vi "test_DL950.vi"() -> ()   [LabVIEW 2019]
uses:
  _ctrl/fgv_DL950.ctl
  _ctrl/rw.ctl
  _ctrl/init-r-stop.ctl
  _ctrl/create-rw-close.ctl
  _ctrl/DL950_config.ctl
panel:
  out "DL950 wfm":waveform(dbl)[](graph)
  out "Waveform":cluster{"l":dbl, "dt":dbl, "Y":dbl[][]}(graph)
  out "n":i32
  out "Read":string
  in  "Qurery":bool
  in  "Write":string
  in  "Disconnection":bool
  in  "Connection":bool
  in  "Get_Items":bool
  in  "Get_Wave":bool
  in  "config":T1={"Timeout"=10000, "Time Div"=12, "Acq Mode"=0, "Record Len"=0, "Record Num"=0, "Start Point"=0, "End Poin"=1000, "Visa"="", "Config Voltage"=[], "Trigger on"=FALSE, "Trigger Level"=0.0, "Reset"=FALSE, "Config Temp"=[], "Trigger Mode"=1, "Trigger Position"=50.0, "Trigger Slope"=0, "Trigger Source "=1, "Start Point (-5.00)"=-5.0, "End Point (5.00)"=5.0} {"End Point (5.00)" format="%.2g"; "Start Point (-5.00)" format="%.2f"; "Trigger Source" items=["", "CH1", "CH2", "CH3", "CH4", "CH5", "CH6", "CH7", "CH8", "CH9", "CH10", "CH11", "CH12", "CH13", "CH14", "CH15", "CH16", "RMATH1", "RMATH2", "RMATH3", "RMATH4", "RMATH5", "RMATH6", "RMATH7", "RMATH8", "RMATH9", "RMATH10", "RMATH11", "RMATH12", "RMATH13", "RMATH14", "RMATH15", "RMATH16"]; "Trigger Slope" items=["Rising", "Falling", "Both"]; "Trigger Position" format="%.1f"; "Trigger Mode" items=["Normal", "Auto", "Auto Level", "Single", "Single(N)", "On Start", "No Set"]; "Config Temp"."Type" items=["K", "E", "J", "T", "L", "U", "N", "R", "S", "B", "W", "Au7fe"]; "Config Temp"."Channel" items=["", "CH1", "CH2", "CH3", "CH4", "CH5", "CH6", "CH7", "CH8", "CH9", "CH10", "CH11", "CH12", "CH13", "CH14", "CH15", "CH16"]; "Trigger Level" format="%.3p"; "Config Voltage"."items" items=["Peak to Peak", "Amplitude", "Max", "Min", "High", "Low", "Average", "Middle", "Rms", "Standard Deviation", "+Overshoot", "-Overshoot", "Rise", "Fall", "Frequency", "Period", "+Width", "-Width", "Duty Cycle", "Pulse Count", "Burst1 Width", "Burst2 Width", "Average Frequency", "Average Period", "Int1TY", "Int2TY"]; "Config Voltage"."Probe" items=["1:1", "2:1", "5:1", "10:1", "20:1", "50:1", "100:1", "200:1", "500:1", "1000:1", "2000:1", "5000:1", "10k:1", "20k:1", "50k:1", "0.1A:1V", "0.2A:1V", "0.5A:1V", "1A:1V", "2A:1V", "5A:1V", "10A:1V", "20A:1V", "50A:1V", "100A:1V", "200A:1V", "250A:1V", "400A:1V", "500A:1V", "1kA:1V", "2kA:1V", "5kA:1V", "10kA:1V", "20kA:1V", "50kA:1V", "NoSet"]; "Config Voltage"."Ch" items=["None", "CH1", "CH2", "CH3", "CH4", "CH5", "CH6", "CH7", "CH8", "CH9", "CH10", "CH11", "CH12", "CH13", "CH14", "CH15", "CH16", "MATH1", "MATH2", "MATH3", "MATH4", "MATH5", "MATH6", "MATH7", "MATH8", "EVENT"]; "Config Voltage"."Coupling" items=["AC", "DC", "Ground", "AC-RMS", "DC-RMS"]; "Config Voltage"."V Div" items=["0.1m", "0.2m", "0.5m", "1m", "2m", "5m", "10m", "20m", "50m", "100m", "200m", "500m", "1", "2", "4", "5", "8", "10", "20", "40", "50", "80", "100", "200", "400", "500", "800", "1k", "2k", "4k", "5k", "8k", "10k", "20k", "25k", "50k", "100k", "250k", "500k", "1000k"]; "Record Len" items=["10k", "25k", "50k", "100k", "250k", "500k", "1M", "2.5M", "5M", "10M", "25M", "50M", "100M", "250M", "500M", "1G", "2G", "4G", "5G", "10G", "20G", "50G"]; "Acq Mode" items=["Normal", "Average", "Envelope"]; "Time Div" items=["100ns", "200ns", "500ns", "1us", "2us", "5us", "10us", "20us", "50us", "100us", "200us", "500us", "1ms", "2ms", "5ms", "10ms", "20ms", "50ms", "100ms", "200ms", "500ms", "1s", "2s", "3s", "4s", "5s", "6s", "10s", "20s", "30s", "1min", "2min", "3min", "4min", "5min", "6min", "10min", "12min", "30min", "1hour", "2hour", "3hour", "4hour", "5hour", "6hour", "8hour", "10hour", "12hour", "1day", "2day", "3day", "4day", "5day"]}
  in  "delay":u32=10
  in  "정지":bool
  # "YOKOGAWA DL950 LabVIEW Instr"
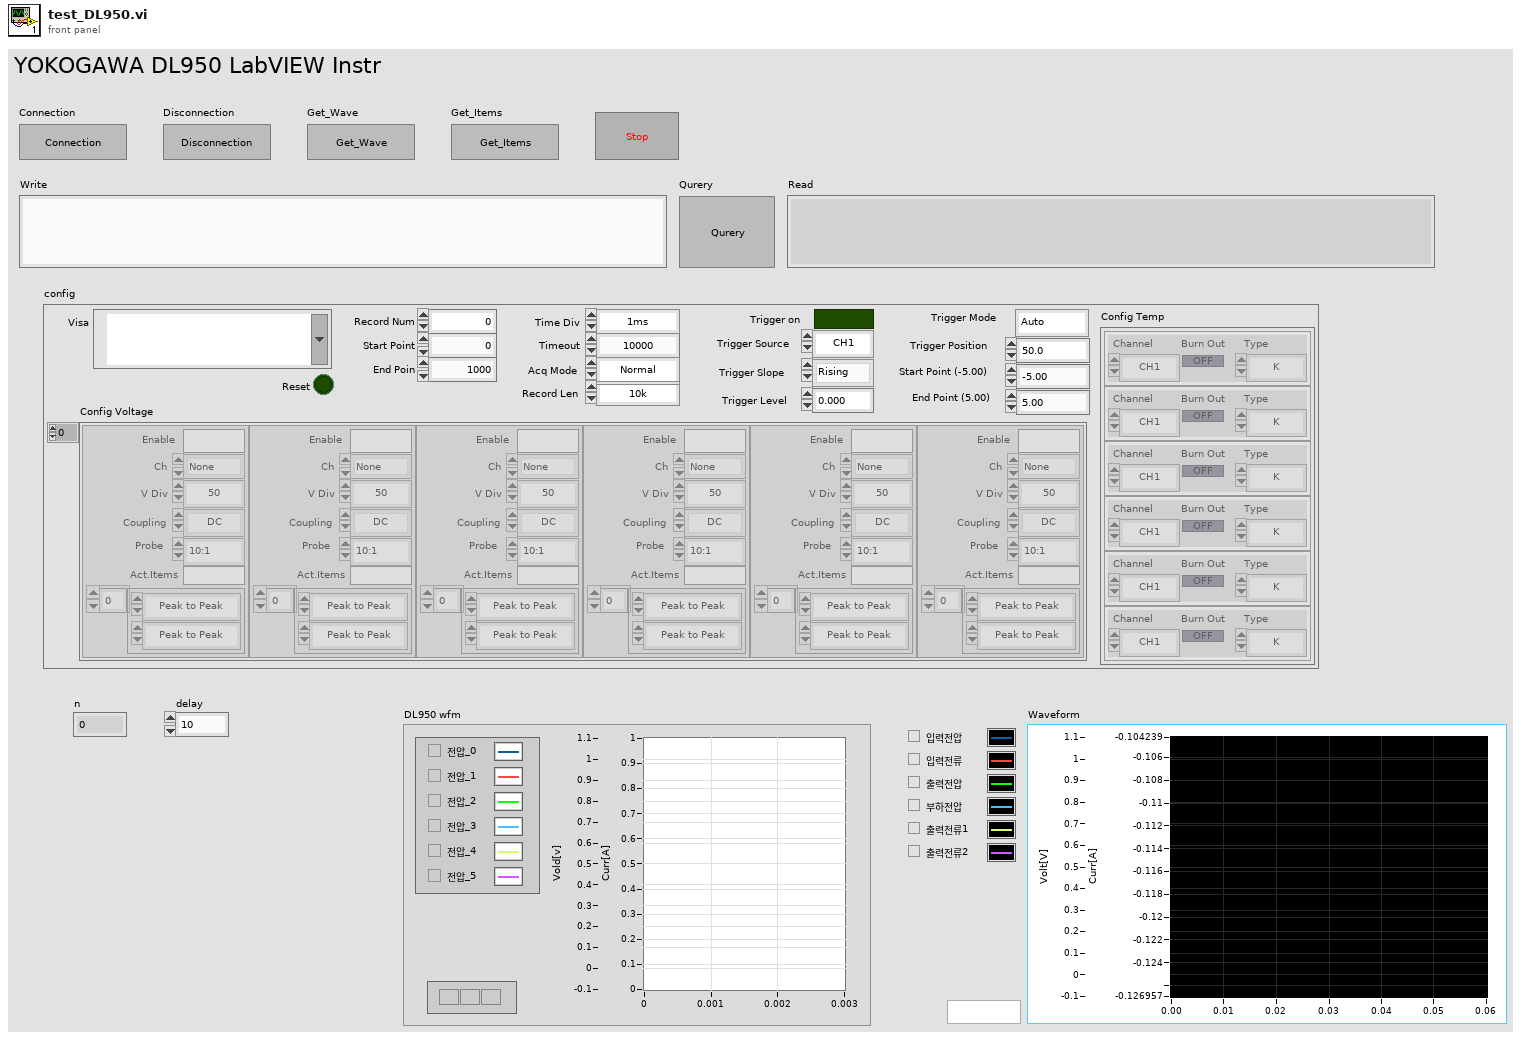
[diagram p1: front panel]
types:
  T1 = typedef "DL950_config.ctl" = cluster{"Timeout":u32, "Time Div":i32, "Acq Mode":i32, "Record Len":i32, "Record Num":i32, "Start Point":i64, "End Poin":i64, "Visa":refnum<visa-resource-name>, "Config Voltage":cluster{"Enable":bool, "Ch":u16, "V Div":i32, "Coupling":i32, "Probe":i32, "Act.Items":bool, "items":i32[]}[], "Trigger on":bool, "Trigger Level":dbl, "Reset":bool, "Config Temp":cluster{"Channel":u16, "Burn Out":bool, " Type ":i32}[], "Trigger Mode":i32, "Trigger Position":dbl, "Trigger Slope":i32, "Trigger Source ":i32, "Start Point (-5.00)":dbl, "End Point (5.00)":dbl}
  T2 = typedef "create-rw-close.ctl" = enum16{"create", "write", "read", "close"}
  T3 = typedef "init-r-stop.ctl" = enum16{"ini", "read", "stop"}
  T4 = typedef "rw.ctl" = enum16{"read", "write"}
  T5 = typedef "fgv_DL950.ctl" = enum16{"init", "config", "Set-NCh", "setapply", "trigger", "read", "time-div", "wave-aquis", "start", "query", "abort", "set_items", "reset_items", "read_items", "percent_rise", "trigger_single", "stop", "close"}
  T6 = typedef "start.ctl" = enum16{"init", "open", "set", "start", "stop", "read", "read_items", "query", "close", "T_single", "reset", "exit"}
  T7 = typedef "DL950_wfms.ctl" = cluster{"wfms":waveform(dbl)[], "Waveform_2":cluster{"t0":dbl, "dt":dbl, "Y":dbl[][]}, "items":dbl[][]}
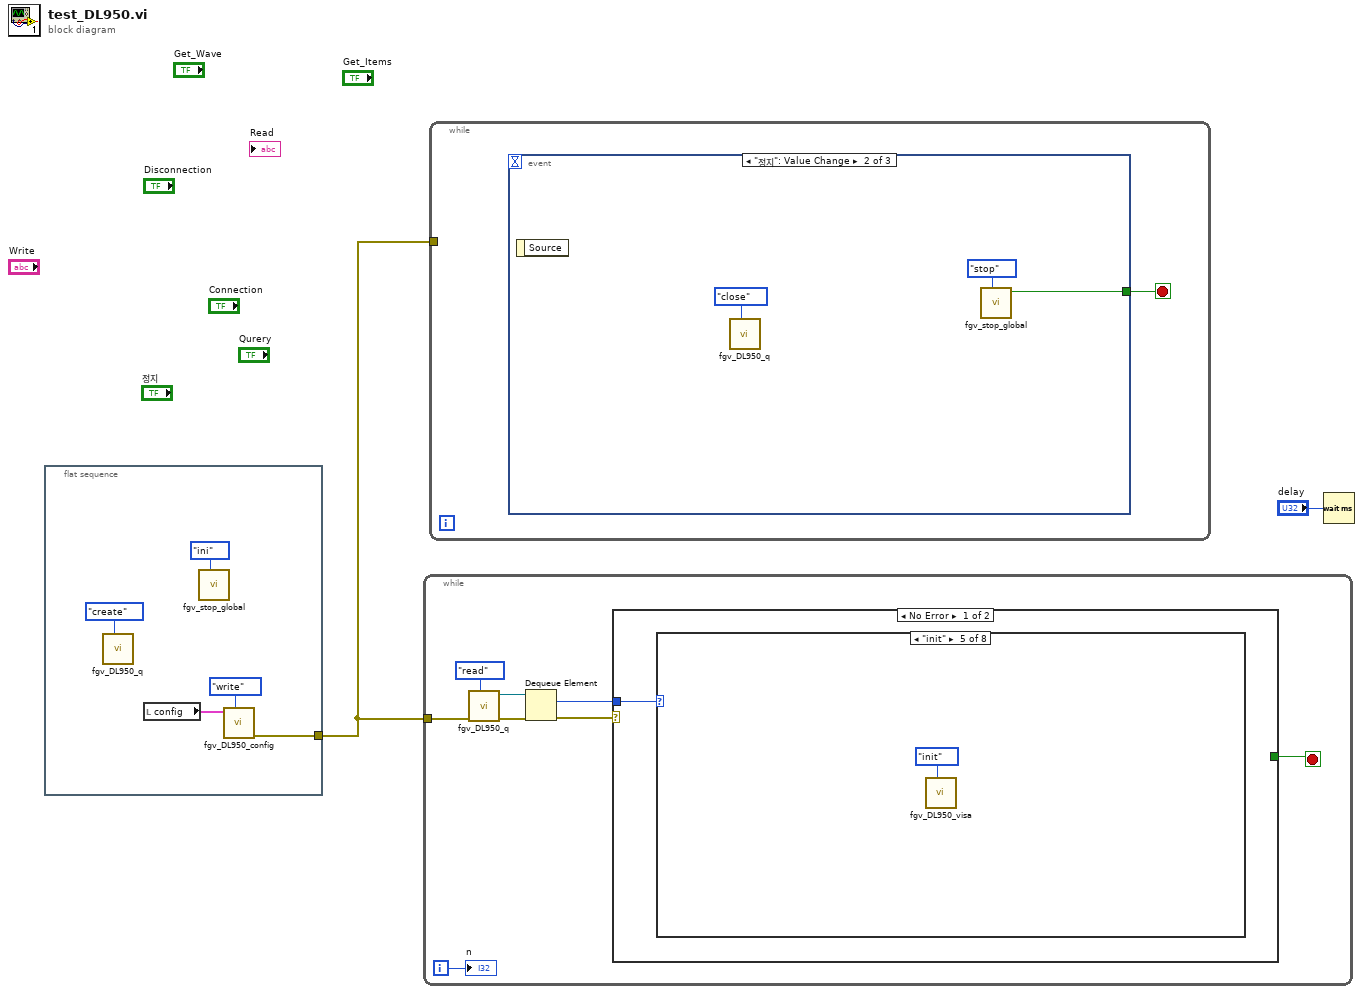
[diagram p0: block diagram]
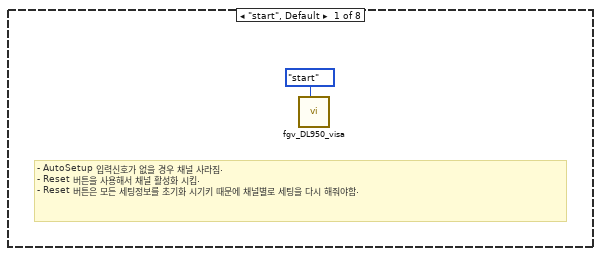
[diagram p2: hidden frame]
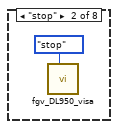
[diagram p3: hidden frame]
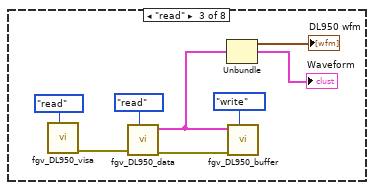
[diagram p4: hidden frame]
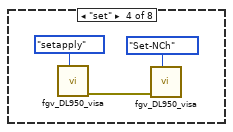
[diagram p5: hidden frame]
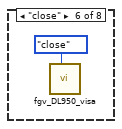
[diagram p6: hidden frame]
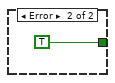
[diagram p9: hidden frame]
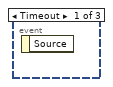
[diagram p10: hidden frame]
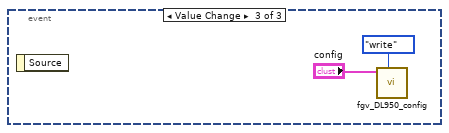
[diagram p11: hidden frame]
diagram:
  n1 = flat-sequence {
    tunnel: [w6] -> w1
    frame #0 {
      n2 = call "fgv_DL950_q.vi"("cmd"=create-rw-close."create") -> ()  [unwired: 9 in, 2 out]
      n3 = local read "config"() -> (w4:T1)
      n4 = call "fgv_stop_global.vi"("cmd"=init-r-stop."ini") -> ()  [unwired: 10 in, 1 out]
      n5 = call "fgv_DL950_config.vi"("cmd"=rw."write", "config"=w4) -> ("error out"=w6:errorcluster)  [unwired: 8 in, 1 out]
    }
  }
  n6 = while {
    tunnel: w1 -> [w8]
    i -> [w9]
    stop <- w10 stop-if-true
    n7 = call "fgv_DL950_q.vi"("cmd"=create-rw-close."read", "error in"=w8) -> ("error out"=w14:errorcluster, "queue out"=w13:refnum<queue>)  [unwired: 8 in]
    n8 = Dequeue Element(queue=w13, error in (no error)=w14) -> (element=w12:T6, error out=w11:errorcluster)  [unwired: 1 in, 2 out]
    n9 = case shown="No Error" w11 {
      tunnel: w12 -> [w16 _]
      tunnel: [_ TRUE ("status")] -> w10
      frame No Error {
        n10 = case shown="\"init\"" w16 {
          frame "start", Default {
            # "- AutoSetup 입력신호가 없을 경우 채널 사라짐.\n- Reset 버튼을 사용해서 채널 활성화 시킴.\n- Reset 버튼은 모든 세팅정보를 초기화 시기키 때문에 채널별로 세팅을 다시 해줘야함."
            n11 = call "fgv_DL950_visa.vi"("cmd"=fgv_DL950."start") -> ()  [unwired: 8 in, 3 out]
          }
          frame "stop" {
            n12 = call "fgv_DL950_visa.vi"("cmd"=fgv_DL950."stop") -> ()  [unwired: 8 in, 3 out]
          }
          frame "read" {
            n13 = call "fgv_DL950_visa.vi"("cmd"=fgv_DL950."read") -> ("error out"=w23:errorcluster)  [unwired: 8 in, 2 out]
            n14 = call "fgv_DL950_data.vi"("cmd"=rw."read", "error in"=w23) -> ("error out"=w22:errorcluster, "DL950 wfm 2"=w20:T7)  [unwired: 8 in]
            n15 = Unbundle(w20) -> ("wfms"=→"DL950 wfm":waveform(dbl)[], "Waveform_2"=→"Waveform":cluster{"t0":dbl, "dt":dbl, "Y":dbl[][]})  [unwired: 1 out]
            n16 = call "fgv_DL950_buffer.vi"("cmd"=create-rw-close."write", "error in"=w22, "DL950 wfm 2"=w20) -> ()  [unwired: 7 in, 2 out]
          }
          frame "set" {
            n17 = call "fgv_DL950_visa.vi"("cmd"=fgv_DL950."setapply") -> ("error out"=w27:errorcluster)  [unwired: 8 in, 2 out]
            n18 = call "fgv_DL950_visa.vi"("cmd"=fgv_DL950."Set-NCh", "error in"=w27) -> ()  [unwired: 7 in, 3 out]
          }
          frame "init" {
            n19 = call "fgv_DL950_visa.vi"("cmd"=fgv_DL950."init") -> ()  [unwired: 8 in, 3 out]
          }
          frame "close" {
            n20 = call "fgv_DL950_visa.vi"("cmd"=fgv_DL950."close") -> ()  [unwired: 8 in, 3 out]
          }
          frame "exit" {
          }
          frame "open" {
          }
        }
      }
      frame Error {
      }
    }
    "n" <- w9
  }
  n21 = while {
    tunnel: w1 -> [_]
    stop <- w33 stop-if-true
    n22 = event shown="[1] \"정지\": Value Change" {
      selector: _ -> [_ _ _]
      dyn-events: _ -> [_ _ _]
      timeout: _ -> [_ _ _]
      tunnel: [_ w35 _] -> w33
      event Timeout {
        n23 = event-data() -> ()  [unwired: 1 in, 1 out]
      }
      event "정지": Value Change {
        n24 = event-data() -> ()  [unwired: 1 in, 1 out]
        n25 = call "fgv_DL950_q.vi"("cmd"=create-rw-close."close") -> ()  [unwired: 9 in, 2 out]
        n26 = call "fgv_stop_global.vi"("cmd"=init-r-stop."stop") -> ("stop"=w35:bool)  [unwired: 10 in]
      }
      event Value Change {
        n27 = event-data() -> ()  [unwired: 1 in, 1 out]
        n28 = call "fgv_DL950_config.vi"("cmd"=rw."write", "config"="config") -> ()  [unwired: 8 in, 2 out]
      }
    }
  }
  n29 = Wait (ms)(milliseconds to wait="delay") -> ()  [unwired: 1 out]
